vi "Save As EDF.vi"(8 "error in (no error)":errorcluster, 10 "iMode":i32, 11 "szPath":string) -> (0 "error out":errorcluster, 2 "function return":u32, 3 "szPath out":string)   [LabVIEW 2014, in "atmcd32d.lvlib"]
doc: "unsigned int WINAPI SaveAsEDF(char * szPath, int iMode);"
uses:
  atmcd32d.lvlib
  atmcd32d.dll
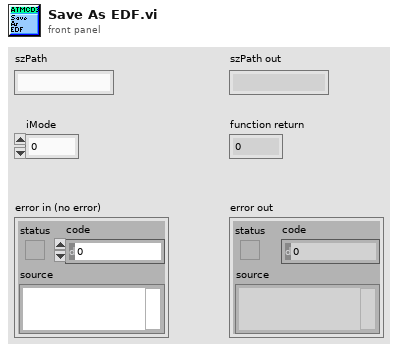
[diagram p1: front panel]
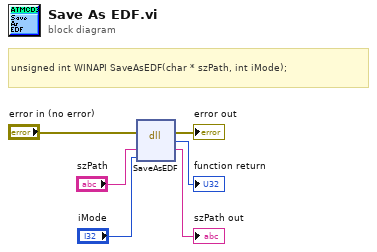
[diagram p0: block diagram]
diagram:
  # "unsigned int WINAPI SaveAsEDF(char * szPath, int iMode);"
  n1 = dll-call lib="C:/Users/Bakir/Documents/Lambda2-Testing/lib/Andorlib/atmcd32d.*" fn="SaveAsEDF"(error in="error in (no error)", "szPath"="szPath", "iMode"="iMode") -> (error out=→"error out":errorcluster, →"function return":u32, "szPath"=→"szPath out":string)  [unwired: 3 in, 1 out]
